vi "Nattify.vi"(6 "Variant in":variant, 7 "Shift Pressed?":bool, 8 "error in":errorcluster, 10 "QD Combo Box Ref":refnum<vi>, 11 "QD Launch VI Ref":refnum<vi>) -> (0 "error out":errorcluster, 4 "Variant out":variant)   [LabVIEW 2020]
doc: "Nattification is the process by which a VI is modified to have the most sensible aesthetics and user-configurable options applied. This means non-terminal view on icons, left-justified subdiagram labels, autogrow disabled on all structures, etc.\n\nDefault Shortcut - [N]"
uses:
  <vilib>/Utility/traverseref.llb/TRef TravTarget.ctl
  <vilib>/Utility/VariantDataType/VariantType.lvlib
  <vilib>/Utility/traverseref.llb/VI Scripting - Traverse.lvlib
panel:
  in  "Undo Name":string="Nattification"
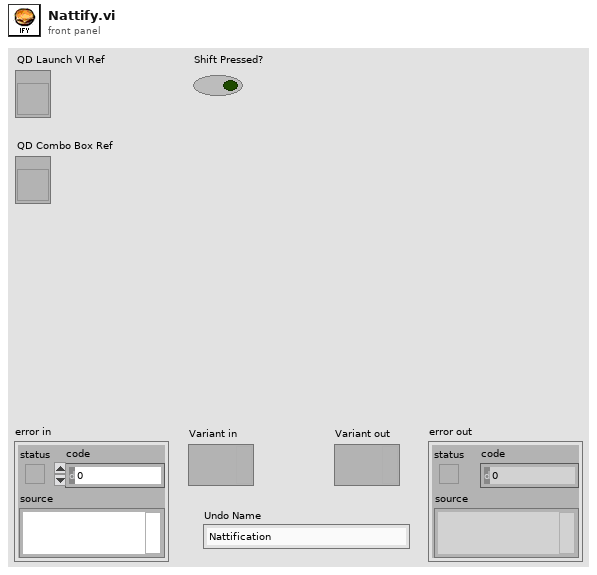
[diagram p1: front panel]
types:
  T1 = typedef "TRef TravTarget.ctl" = enum16{"FP", "BD", "Other"}
  T2 = enum16{"Auto Error Handling", "Autogrow", "Front Panel Color", "Icon View", "Move Error Wires Back", "Remove (no error)", "Subdiagram Label Justify", "Terminal Labels on Side", "Terminal Labels Transparent", "Arrange Windows"}
  T3 = typedef "LVRectTypeDef.ctl" = cluster{"Left":i16, "Top":i16, "Right":i16, "Bottom":i16}
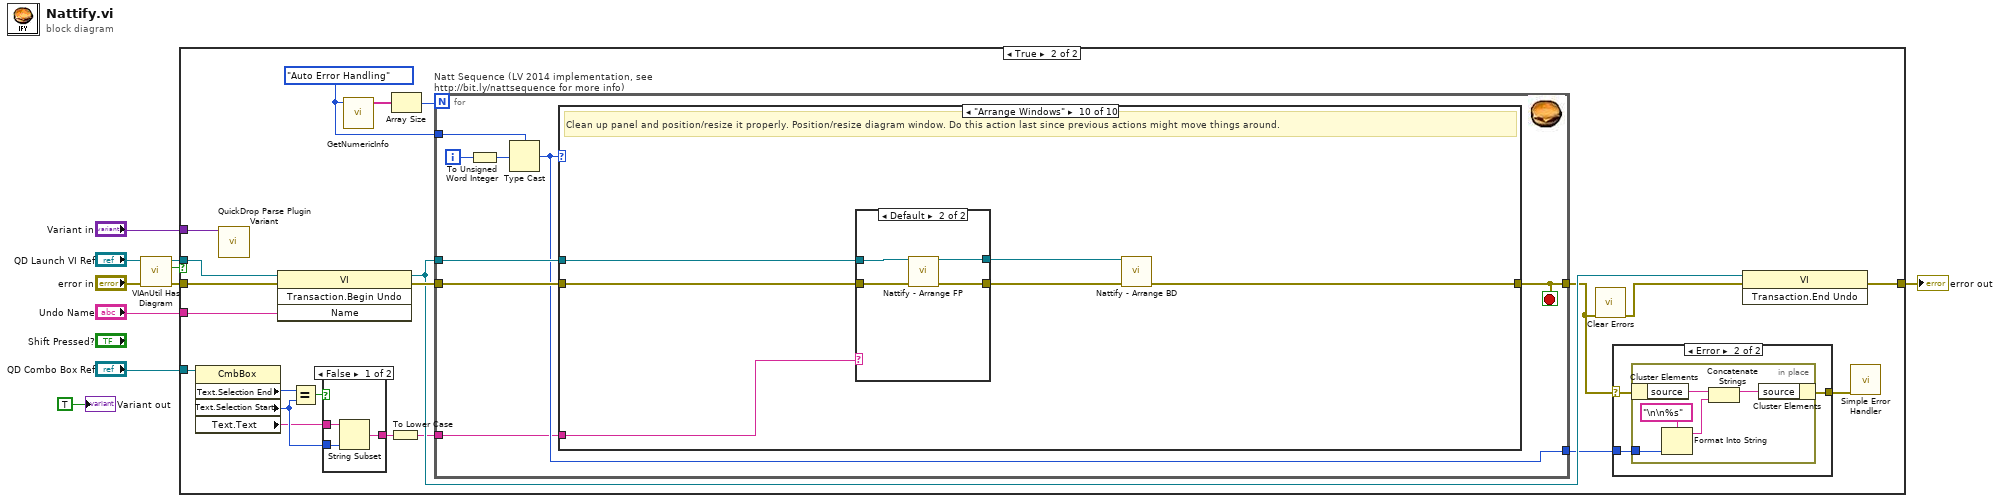
[diagram p0: block diagram]
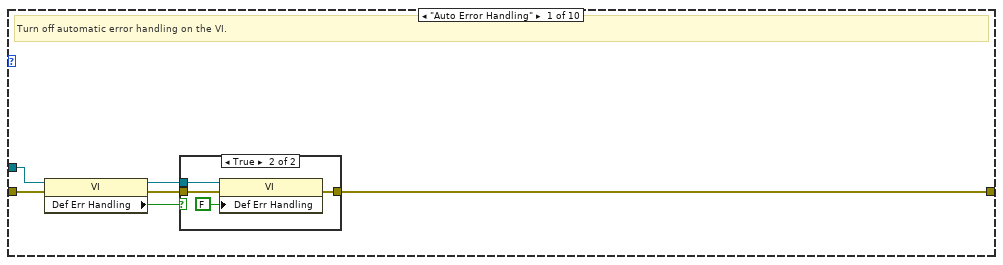
[diagram p5: hidden frame]
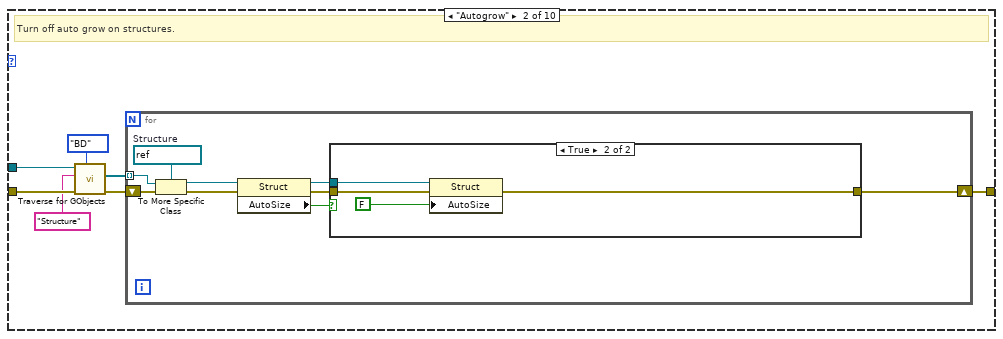
[diagram p7: hidden frame]
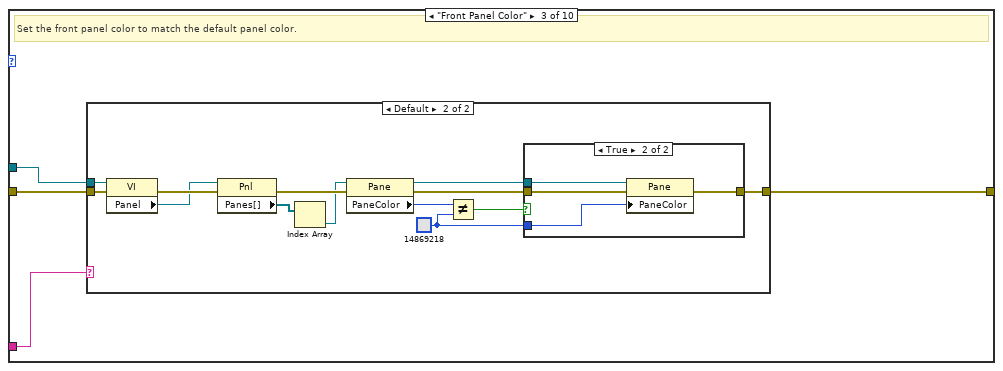
[diagram p9: hidden frame]
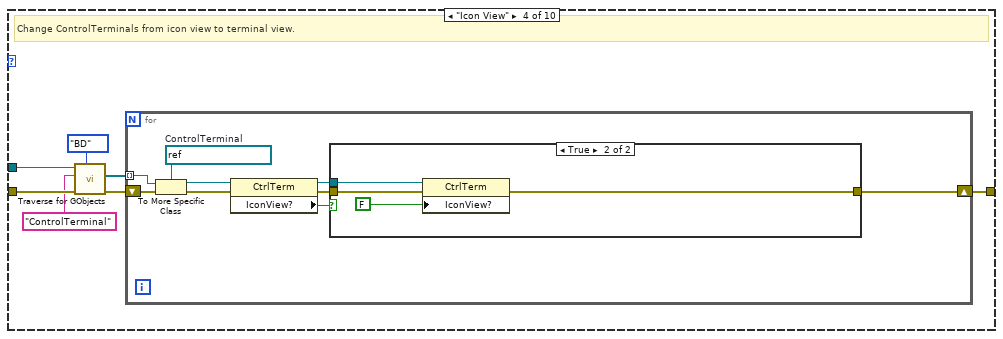
[diagram p12: hidden frame]
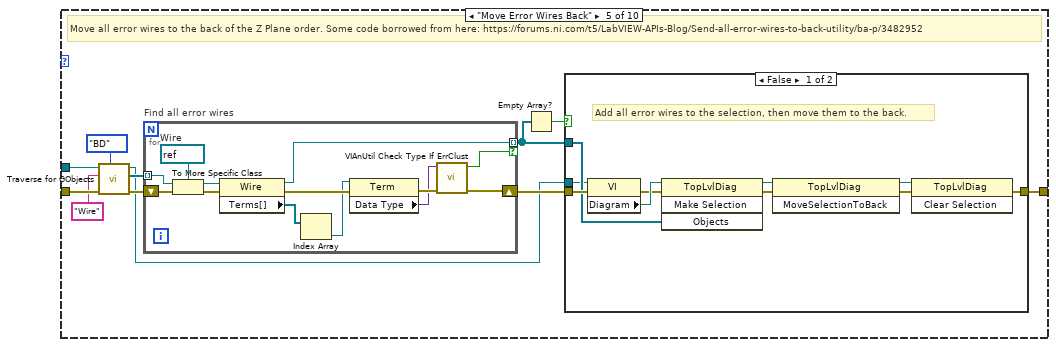
[diagram p14: hidden frame]
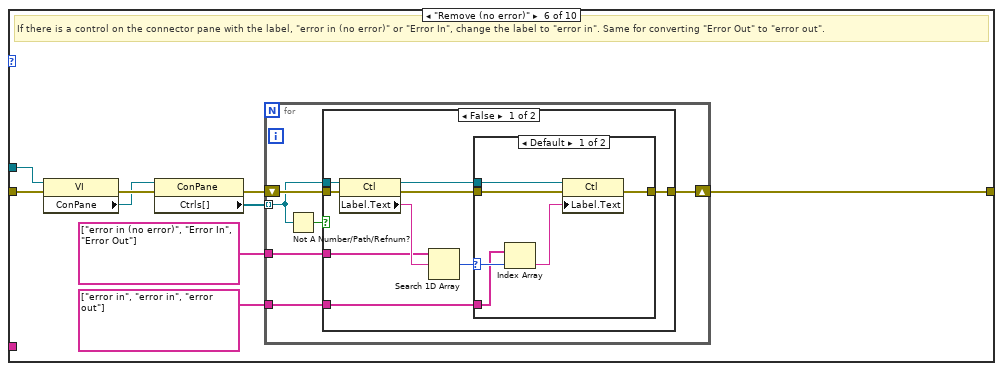
[diagram p16: hidden frame]
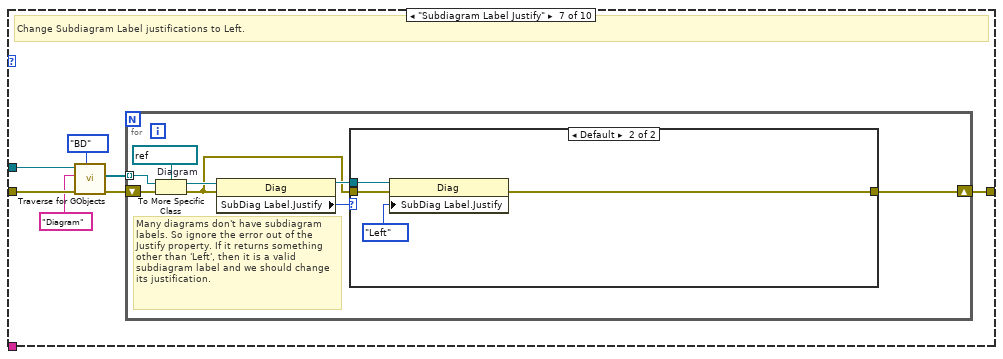
[diagram p19: hidden frame]
diagram:
  n1 = call <vilib>:"VIAnUtil Has Diagram.vi"("error in (no error)"="error in", "VI in"="QD Launch VI Ref") -> ("error out"=w5:errorcluster, "Has Diag?"=w2:bool, "VI out"=w3:refnum<vi>)  [unwired: 4 in, 3 out]
  n2 = case shown="True" w2 {
    tunnel: [w11 w32] -> w10
    tunnel: "Variant in" -> [_ w31]
    tunnel: "Undo Name" -> [_ w30]
    tunnel: w5 -> [w11 w24]
    tunnel: w3 -> [_ w23]
    tunnel: "QD Combo Box Ref" -> [_ w13]
    frame False {
      # "This plugin doesn't provide much useful functionaity for VIs that don't have diagrams, so just no-op for those."
    }
    frame True {
      w26 = T2."Auto Error Handling"
      n3 = property on="Property Node" class="CmbBox"(reference=w13) -> ("Text.Selection End"=w18:u32, "Text.Selection Start"=w16:u32, "Text.Text"=w15:string)  [unwired: 1 in, 2 out]
      n4 = call <vilib>:"QuickDrop Parse Plugin Variant.vi"("QDKS Variant in"=w31) -> ()  [unwired: 12 in, 3 out]
      n5 = invoke class="VI" method="Transaction.Begin Undo"(reference=w23, error in=w24, "Name"=w30) -> (reference out=w25:refnum<vi>, error out=w29:errorcluster)  [unwired: 1 in, 2 out]
      n6 = Equal?(x=w18, y=w16) -> (x = y?=w17:bool)
      n7 = case shown="False" w17 {
        tunnel: [w35 w36] -> w14
        tunnel: w16 -> [w34 _]
        tunnel: w15 -> [w33 w36]
        frame False {
          n8 = String Subset(string=w33, length (rest)=w34) -> (substring=w35:string)  [unwired: 1 out]
        }
        frame True {
        }
      }
      n9 = call <vilib>:"GetNumericInfo.vi"("Variant"=w26) -> ("EnumNames"=w27:string[])  [unwired: 7 in, 3 out]
      n10 = To Lower Case(string=w14) -> (all lower case string=w12:string)
      n11 = Array Size(array=w27) -> (size(s)=w28:i32)
      n12 = for "Natt Sequence (LV 2014 implementation, see http://bit.ly/nattsequence for more info)" {
        N: w28 -> [_]
        tunnel: w26 -> [w51]
        tunnel: w29 -> [w50]
        tunnel: [w49] -> w21
        tunnel: w25 -> [w48]
        tunnel: [w47] -> w19
        tunnel: w12 -> [w46]
        i -> [w53]
        stop <- w49 stop-if-true
        n13 = To Unsigned Word Integer(number=w53) -> (unsigned 16bit integer=w52:u16)
        n14 = Type Cast(type=w51, x=w52) -> (*(type *) &x=w47:T2)
        n15 = case shown="\"Arrange Windows\"" w47 {
          tunnel: w50 -> [w59 w71 w89 w115 w140 w173 w203 w223 w252 w269]
          tunnel: [w54 w65 w87 w109 w131 w166 w197 w217 w251 w268] -> w49
          tunnel: w48 -> [w58 w70 w88 w114 w139 w172 w202 w222 w253 w266]
          tunnel: w46 -> [_ _ w86 _ _ _ _ _ _ w267]
          frame "Auto Error Handling" {
            # "Turn off automatic error handling on the VI."
            n16 = property class="VI"(reference=w58, error in=w59) -> (reference out=w55:refnum<vi>, error out=w57:errorcluster, "Def Err Handling"=w56:bool)
            n17 = case shown="True" w56 {
              tunnel: w57 -> [w60 w63]
              tunnel: w55 -> [_ w64]
              tunnel: [w60 w61] -> w54
              frame False {
              }
              frame True {
                n18 = property class="VI"(reference=w64, error in=w63, "Def Err Handling"=FALSE ("Automatic Error Handling")) -> (error out=w61:errorcluster)  [unwired: 1 out]
              }
            }
          }
          frame "Autogrow" {
            # "Turn off auto grow on structures."
            n19 = call <vilib>:"Traverse for GObjects.vi"("Traverse Target"=TRef_TravTarget."BD", "error in (no error)"=w71, "Class Name"="Structure", "VI Refnum"=w70) -> ("error out"=w67:errorcluster, "References"=w66:refnum<vi>[])  [unwired: 4 in, 2 out]
            n20 = for {
              shift-right: [w75] -> w65
              shift-left: w67 -> [w80]
              tunnel: w66 -> [w79] mode=indexing
              w78 = refnum<vi> refnum  # Structure
              n21 = To More Specific Class(target class=w78, reference=w79, error in=w80) -> (specific class reference=w77:refnum<vi>, error out=w76:errorcluster)
              n22 = property class="Struct"(reference=w77, error in=w76) -> (reference out=w73:refnum<vi>, error out=w74:errorcluster, "AutoSize"=w72:bool)
              n23 = case shown="True" w72 {
                tunnel: [w81 w84] -> w75
                tunnel: w74 -> [w81 w85]
                tunnel: w73 -> [_ w83]
                frame False {
                }
                frame True {
                  n24 = property class="Struct"(reference=w83, error in=w85, "AutoSize"=FALSE ("Icon View?")) -> (error out=w84:errorcluster)  [unwired: 1 out]
                }
              }
            }
          }
          frame "Front Panel Color" {
            # "Set the front panel color to match the default panel color."
            n25 = case shown="Default" w86 {
              tunnel: w89 -> [w90 w103]
              tunnel: w88 -> [_ w102]
              tunnel: [w90 w91] -> w87
              frame "p" {
                # "Don't change panel color if 'p' was typed"
              }
              frame Default {
                w95 = u32 14869218
                n26 = property class="VI"(reference=w102, error in=w103) -> (error out=w101:errorcluster, "Panel"=w100:refnum<vi>)  [unwired: 1 out]
                n27 = property class="Pnl"(reference=w100, error in=w101) -> (error out=w98:errorcluster, "Panes[]"=w99:refnum<vi>[])  [unwired: 1 out]
                n28 = Index Array(array=w99) -> (element=w97:refnum<vi>)  [unwired: 1 in]
                n29 = property class="Pane"(reference=w97, error in=w98) -> (reference out=w94:refnum<vi>, error out=w93:errorcluster, "PaneColor"=w92:u32)
                n30 = Not Equal?(x=w92, y=w95) -> (x != y?=w96:bool)
                n31 = case shown="True" w96 {
                  tunnel: [w104 w107] -> w91
                  tunnel: w93 -> [w104 w108]
                  tunnel: w94 -> [_ w106]
                  tunnel: w95 -> [_ w105]
                  frame False {
                  }
                  frame True {
                    n32 = property class="Pane"(reference=w106, error in=w108, "PaneColor"=w105) -> (error out=w107:errorcluster)  [unwired: 1 out]
                  }
                }
              }
            }
          }
          frame "Icon View" {
            # "Change ControlTerminals from icon view to terminal view."
            n33 = call <vilib>:"Traverse for GObjects.vi"("Traverse Target"=TRef_TravTarget."BD", "error in (no error)"=w115, "Class Name"="ControlTerminal", "VI Refnum"=w114) -> ("error out"=w111:errorcluster, "References"=w110:refnum<vi>[])  [unwired: 4 in, 2 out]
            n34 = for {
              shift-right: [w119] -> w109
              shift-left: w111 -> [w124]
              tunnel: w110 -> [w123] mode=indexing
              w122 = refnum<vi> refnum  # ControlTerminal
              n35 = To More Specific Class(target class=w122, reference=w123, error in=w124) -> (specific class reference=w121:refnum<vi>, error out=w120:errorcluster)
              n36 = property class="CtrlTerm"(reference=w121, error in=w120) -> (reference out=w117:refnum<vi>, error out=w118:errorcluster, "IconView?"=w116:bool)
              n37 = case shown="True" w116 {
                tunnel: [w125 w128] -> w119
                tunnel: w118 -> [w125 w129]
                tunnel: w117 -> [_ w127]
                frame False {
                }
                frame True {
                  n38 = property class="CtrlTerm"(reference=w127, error in=w129, "IconView?"=FALSE ("Icon View?")) -> (error out=w128:errorcluster)  [unwired: 1 out]
                }
              }
            }
          }
          frame "Move Error Wires Back" {
            # "Move all error wires to the back of the Z Plane order. Some code borrowed from here: https://forums.ni.com/t5/LabVIEW-APIs-Blog/Send-all-error-wires-to-back-utility/ba-p/3482952"
            n39 = call <vilib>:"Traverse for GObjects.vi"("Traverse Target"=TRef_TravTarget."BD", "error in (no error)"=w140, "Class Name"="Wire", "VI Refnum"=w139) -> ("error out"=w136:errorcluster, "References"=w135:refnum<vi>[], "dup VI Refnum"=w130:refnum<vi>)  [unwired: 4 in, 1 out]
            n40 = for "Find all error wires" {
              tunnel: w135 -> [w162] mode=indexing
              shift-right: [w152] -> w133
              shift-left: w136 -> [w164]
              tunnel: [w154] -> w132 mode=indexing if=w153
              w160 = refnum<vi> refnum  # Wire
              n41 = To More Specific Class(target class=w160, reference=w162, error in=w164) -> (specific class reference=w161:refnum<vi>, error out=w163:errorcluster)
              n42 = property class="Wire"(reference=w161, error in=w163) -> (reference out=w154:refnum<vi>, error out=w158:errorcluster, "Terms[]"=w159:refnum<vi>[])
              n43 = Index Array(array=w159) -> (element=w157:refnum<vi>)  [unwired: 1 in]
              n44 = property class="Term"(reference=w157, error in=w158) -> (error out=w156:errorcluster, "Data Type"=w155:variant)  [unwired: 1 out]
              n45 = call <vilib>:"VIAnUtil Check Type If ErrClust.vi"("error in (no error)"=w156, "Data In"=w155) -> ("error out"=w152:errorcluster, "IsErrClust?"=w153:bool)  [unwired: 8 in]
            }
            n46 = Empty Array?(array=w132) -> (empty?=w134:bool)
            n47 = case shown="False" w134 {
              tunnel: w133 -> [w147 w151]
              tunnel: w132 -> [w144 _]
              tunnel: [w142 w151] -> w131
              tunnel: w130 -> [w143 _]
              frame False {
                # "Add all error wires to the selection, then move them to the back."
                n48 = property class="VI"(reference=w143, error in=w147) -> (error out=w146:errorcluster, "Diagram"=w148:refnum<vi>)  [unwired: 1 out]
                n49 = invoke class="TopLvlDiag" method="Make Selection"(reference=w148, error in=w146, "Objects"=w144) -> (reference out=w150:refnum<vi>, error out=w149:errorcluster)  [unwired: 1 in, 2 out]
                n50 = invoke class="TopLvlDiag" method="MoveSelectionToBack"(reference=w150, error in=w149) -> (reference out=w141:refnum<vi>, error out=w145:errorcluster)  [unwired: 1 in, 1 out]
                n51 = invoke class="TopLvlDiag" method="Clear Selection"(reference=w141, error in=w145) -> (error out=w142:errorcluster)  [unwired: 1 in, 2 out]
              }
              frame True {
                # "No error wires on the diagram."
              }
            }
          }
          frame "Remove (no error)" {
            # "If there is a control on the connector pane with the label, \"error in (no error)\" or \"Error In\", change the label to \"error in\". Same for converting \"Error Out\" to \"error out\"."
            n52 = property class="VI"(reference=w172, error in=w173) -> (error out=w171:errorcluster, "ConPane"=w170:refnum<vi>)  [unwired: 1 out]
            n53 = property class="ConPane"(reference=w170, error in=w171) -> (error out=w169:errorcluster, "Ctrls[]"=w168:refnum<vi>[])  [unwired: 1 out]
            n54 = for {
              shift-right: [w177] -> w166
              shift-left: w169 -> [w179]
              tunnel: w168 -> [w175] mode=indexing
              tunnel: string[] ["error in (no error)", "Error In", "Error Out"] -> [w178]
              tunnel: string[] ["error in", "error in", "error out"] -> [w176]
              n55 = Not A Number/Path/Refnum?(number/path/refnum=w175) -> (NaN/Path/Refnum?=w174:bool)
              n56 = case shown="False" w174 {
                tunnel: w179 -> [w188 w196]
                tunnel: w175 -> [w187 _]
                tunnel: w178 -> [w185 _]
                tunnel: [w182 w196] -> w177
                tunnel: w176 -> [w180 _]
                frame False {
                  n57 = property class="Ctl"(reference=w187, error in=w188) -> (reference out=w181:refnum<vi>, error out=w184:errorcluster, "Label.Text"=w186:string)
                  n58 = Search 1D Array(1D array=w185, element=w186) -> (index of element=w183:i32)  [unwired: 1 in]
                  n59 = case shown="Default" w183 {
                    selector: w183 -> [w191 _]
                    tunnel: w184 -> [w192 w195]
                    tunnel: [w193 w195] -> w182
                    tunnel: w181 -> [w194 _]
                    tunnel: w180 -> [w190 _]
                    frame Default {
                      n60 = Index Array(array=w190, index=w191) -> (element=w189:string)
                      n61 = property class="Ctl"(reference=w194, error in=w192, "Label.Text"=w189) -> (error out=w193:errorcluster)  [unwired: 1 out]
                    }
                    frame -1 {
                    }
                  }
                }
                frame True {
                  # "Empty spot on the conpane, ignore it."
                }
              }
            }
          }
          frame "Subdiagram Label Justify" {
            # "Change Subdiagram Label justifications to Left."
            n62 = call <vilib>:"Traverse for GObjects.vi"("Traverse Target"=TRef_TravTarget."BD", "error in (no error)"=w203, "Class Name"="Diagram", "VI Refnum"=w202) -> ("error out"=w199:errorcluster, "References"=w198:refnum<vi>[])  [unwired: 4 in, 2 out]
            n63 = for {
              shift-right: [w204] -> w197
              shift-left: w199 -> [w211]
              tunnel: w198 -> [w210] mode=indexing
              w209 = refnum<vi> refnum  # Diagram
              # "Many diagrams don't have subdiagram labels. So ignore the error out of the Justify property. If it returns something other than 'Left', then it is a valid subdiagram label and we should change its justification."
              n64 = To More Specific Class(target class=w209, reference=w210, error in=w211) -> (specific class reference=w208:refnum<vi>, error out=w205:errorcluster)
              n65 = property class="Diag"(reference=w208, error in=w205) -> (reference out=w206:refnum<vi>, "SubDiag Label.Justify"=w207:enum16{"Left", "Center", "Right"})  [unwired: 1 out]
              n66 = case shown="Default" w207 {
                tunnel: w206 -> [_ w216]
                tunnel: w205 -> [w212 w215]
                tunnel: [w212 w214] -> w204
                frame "Left" {
                }
                frame Default {
                  n67 = property class="Diag"(reference=w216, error in=w215, "SubDiag Label.Justify"=enum16{"Left", "Center", "Right"}."Left" ("Subdiagram Label.Justification")) -> (error out=w214:errorcluster)  [unwired: 1 out]
                }
              }
            }
          }
          frame "Terminal Labels on Side" {
            # "Move control and indicator terminal labels to the sides. Code borrowed from here: resource\\dialog\\QuickDrop\\plugins\\Move Labels.vi"
            n68 = call <vilib>:"Traverse for GObjects.vi"("Traverse Target"=TRef_TravTarget."BD", "error in (no error)"=w223, "Class Name"="ControlTerminal", "VI Refnum"=w222) -> ("error out"=w218:errorcluster, "References"=w219:refnum<vi>[])  [unwired: 4 in, 2 out]
            n69 = for {
              shift-right: [w240] -> w217
              shift-left: w218 -> [w239]
              tunnel: w219 -> [w231] mode=indexing
              w230 = refnum<vi> refnum  # ControlTerminal
              n70 = To More Specific Class(target class=w230, reference=w231, error in=w239) -> (specific class reference=w228:refnum<vi>, error out=w229:errorcluster)
              n71 = property class="CtrlTerm"(reference=w228, error in=w229) -> (error out=w227:errorcluster, "MasterRect"=w225:T3, "Label"=w226:refnum<vi>, "IsSource"=w224:bool)  [unwired: 1 out]
              n72 = property class="Txt" props=["Bounds Rect", "Justify"](reference=w226, error in=w227) -> (reference out=w238:refnum<vi>, error out=w236:errorcluster, "Bounds Rect"=w235:T3)  [unwired: 1 out]
              n73 = case shown="False" w224 {
                tunnel: w225 -> [w243 w250]
                tunnel: w235 -> [_ w248]
                tunnel: [w242 w245] -> w234
                tunnel: [enum16{"Left", "Center", "Right"}."Left" ("Justification") enum16{"Left", "Center", "Right"}."Right" ("Justification")] -> w233
                frame False {
                  n74 = Unbundle By Name(w243) -> ("Right"=w242:i16)
                }
                frame True {
                  n75 = Unbundle By Name(w250) -> ("Left"=w249:i16)
                  n76 = Unbundle By Name(w248) -> ("Right"=w247:i16, "Left"=w246:i16)
                  n77 = Compound Arithmetic op=ADD(w249, invert w247, w246) -> (w245:i16)
                }
              }
              n78 = Unbundle By Name(w225) -> ("Top"=w237:i16)
              n79 = property class="Txt"(reference=w238, error in=w236, "Top"=w237, "Left"=w234, "Justify"=w233, "Visible"=TRUE) -> (error out=w240:errorcluster)  [unwired: 1 out]
            }
          }
          frame "Terminal Labels Transparent" {
            # "Make all control terminal labels have transparent backgrounds."
            n80 = call <vilib>:"Traverse for GObjects.vi"("Traverse Target"=TRef_TravTarget."BD", "error in (no error)"=w252, "Class Name"="ControlTerminal", "VI Refnum"=w253) -> ("error out"=w255:errorcluster, "References"=w254:refnum<vi>[])  [unwired: 4 in, 2 out]
            n81 = for {
              shift-right: [w259] -> w251
              shift-left: w255 -> [w264]
              tunnel: w254 -> [w263] mode=indexing
              w258 = u32 16777216
              w262 = refnum<vi> refnum  # ControlTerminal
              n82 = To More Specific Class(target class=w262, reference=w263, error in=w264) -> (specific class reference=w261:refnum<vi>, error out=w260:errorcluster)
              n83 = property class="CtrlTerm"(reference=w261, error in=w260, "Label.BG Color"=w258, "Label.FG Color"=w258, "Label.BGColor"=w258) -> (error out=w259:errorcluster)  [unwired: 1 out]
            }
          }
          frame "Arrange Windows" {
            # "Clean up panel and position/resize it properly. Position/resize diagram window. Do this action last since previous actions might move things around."
            n84 = case shown="Default" w267 {
              tunnel: [w271 w275] -> w270
              tunnel: w269 -> [w271 w274]
              tunnel: [w272 w273] -> w265
              tunnel: w266 -> [w272 w273]
              frame "p" {
                # "don't arrange panel if 'p' was typed"
              }
              frame Default {
                n85 = call "Nattify - Arrange FP.vi"("VI in"=w273, "error in"=w274) -> ("error out"=w275:errorcluster)  [unwired: 12 in, 1 out]
              }
            }
            n86 = call "Nattify - Arrange BD.vi"("VI in"=w265, "error in"=w270) -> ("error out"=w268:errorcluster)  [unwired: 13 in]
          }
        }
      }
      n87 = call <vilib>:"Clear Errors.vi"("error in (no error)"=w21) -> ("error out"=w22:errorcluster)  [unwired: 5 in, 1 out]
      n88 = case shown="Error" w21 {
        selector: w21 -> [w37 w40]
        tunnel: [w37 w39] -> w20
        tunnel: w19 -> [_ w38]
        frame No Error {
        }
        frame Error {
          n89 = in-place {
            in-place-border: w38 -> [w41]
            n90 = in-place-cluster #1(w40) -> ("source"=w45:string)
            n91 = Format Into String(format string="\n\n%s", w41) -> (resulting string=w43:string)  [unwired: 2 in, 1 out]
            n92 = Concatenate Strings(w45, w43) -> (w44:string)
            n93 = in-place-cluster #1("source"=w44) -> (w39:errorcluster)
          }
        }
      }
      n94 = invoke class="VI" method="Transaction.End Undo"(reference=w25, error in=w22) -> (error out=w32:errorcluster)  [unwired: 1 in, 2 out]
      n95 = call <vilib>:"Simple Error Handler.vi"("error in (no error)"=w20) -> ()  [unwired: 4 in, 5 out]
    }
  }
  "error out" <- w10
  "Variant out" <- TRUE
